vi "Add.vi"(8 "error in (no error)":errorcluster, 9 "Add Options":T1, 10 "Files to Add":path[](array[path]), 11 "Git Implementation in":refnum<class "Git Implementation.lvclass">) -> (0 "error out":errorcluster, 2 "Status Message":string, 3 "Git Implementation out":refnum<class "Git Implementation.lvclass">)   [LabVIEW 2017, in "Git Implementation.lvclass"]
doc: "Add specific files from the working tree to the index (stage the files).\nThis operation prepares the index for an upcoming Commit operation."
uses:
  Git Implementation.lvclass
  Add Options.ctl
  <vilib>/Utility/error.llb/Error Cluster From Error Code.vi
  <vilib>/ErrorRing/Error Ring.xnode
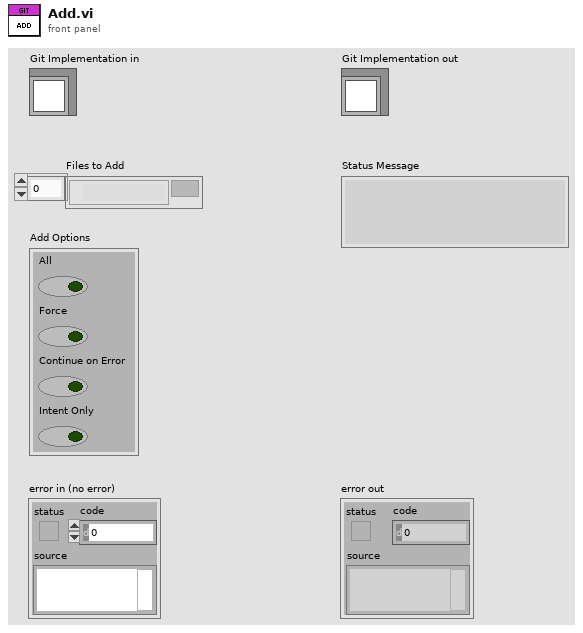
[diagram p1: front panel]
types:
  T1 = typedef "Git Implementation.lvclass/Add Options.ctl" = cluster{"All":bool, "Force":bool, "Continue on Error":bool, "Intent Only":bool}
  T2 = typedef "Git Implementation.lvclass/CMD Return.ctl" = cluster{"StdOut":string, "StdErr":string, "Return Code":i32}
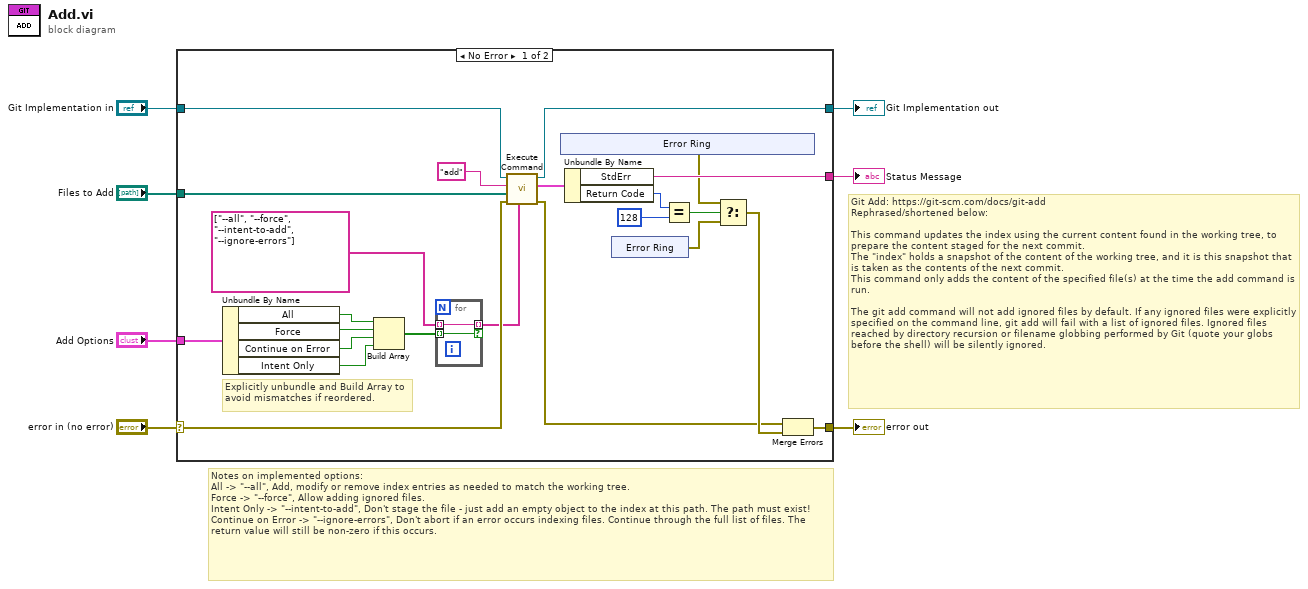
[diagram p0: block diagram]
diagram:
  # "Notes on implemented options:\nAll -> \"--all\", Add, modify or remove index entries as needed to match the working tree.\nForce -> \"--force\", Allow adding ignored files.\nIntent Only -> \"--intent-to-add\", Don't stage the file - just add an empty object to the index at this path. The path must exist!\nContinue on Error -> \"--ignore-errors\", Don't abort if an error occurs indexing files. Continue through the full list of files. The return value will still be non-zero if this occurs."
  # "Git Add: https://git-scm.com/docs/git-add\nRephrased/shortened below:\n\nThis command updates the index using the current content found in the working tree, to prepare the content staged for the next commit.\nThe \"index\" holds a snapshot of the content of the working tree, and it is this snapshot that is taken as the contents of the next commit.\nThis command only adds the content of the specified file(s) at the time the add command is run.\n\nThe git add command will not add ignored files by default. If any ignored files were explicitly specified on the command line, git add will fail with a list of ignored files. Ignored files reached by directory recursion or filename globbing performed by Git (quote your globs before the shell) will be silently ignored."
  n1 = case shown="No Error" "error in (no error)" {
    selector: "error in (no error)" -> [w20 w39]
    tunnel: [w8 w39] -> w6
    tunnel: [w21 w38] -> w4
    tunnel: "Git Implementation in" -> [w22 w38]
    tunnel: "Files to Add" -> [w17 _]
    tunnel: "Add Options" -> [w29 _]
    tunnel: [w14 _] -> w1
    frame No Error {
      # "Explicitly unbundle and Build Array to avoid mismatches if reordered."
      n2 = Unbundle By Name(w29) -> ("All"=w28:bool, "Force"=w27:bool, "Continue on Error"=w26:bool, "Intent Only"=w25:bool)
      n3 = Build Array(w28, w27, w26, w25) -> (w24:bool[])
      n4 = for {
        tunnel: w24 -> [w36] mode=indexing
        tunnel: string[] ["--all", "--force", "--intent-to-add", "--ignore-errors"] -> [w37] mode=indexing
        tunnel: [w37] -> w18 mode=indexing if=w36
      }
      n5 = call "Execute Command.vi"("Arguments"=w18, "error in (no error)"=w20, "File Paths"=w17, "Command"="add", "Git Implementation in"=w22) -> ("error out"=w19:errorcluster, "CMD Return"=w15:T2, "Git Implementation out"=w21:refnum<class "Git Implementation.lvclass">)  [unwired: 4 in]
      n6 = xnode "Error Ring"() -> ("error out"=w10:errorcluster)
      n7 = Unbundle By Name(w15) -> ("StdErr"=w14:string, "Return Code"=w13:i32)
      n8 = xnode "Error Ring"() -> ("error out"=w9:errorcluster)
      n9 = Equal?(x=w13, y=128) -> (x = y?=w11:bool)
      n10 = Select(t=w10, s=w11, f=w9) -> (s? t:f=w30:errorcluster)
      n11 = Merge Errors(w19, w30) -> (w8:errorcluster)
    }
    frame Error {
    }
  }
  "error out" <- w6
  "Git Implementation out" <- w4
  "Status Message" <- w1
